vi "RC_STM_Client 3.vi"() -> ()   [LabVIEW 2019, in "RemoteControl.STM.lvclass"]
uses:
  RemoteControl.STM.lvclass
  RemoteControl/RemoteControl.lvclass
  <userlib>/_OpenG.lib/numeric/numeric.llb/Random Number Within Range - I32__ogtk.vi
  <userlib>/_OpenG.lib/error/error.llb/Filter Error Codes (Array)__ogtk.vi
panel:
  in  "milliseconds to wait":u32
  out "time (1 message) (ms)":u32
  out "startup time (ms)":u32
  out "messsages/s":dbl
  in  "remote port":u16=6341
  in  "address":string
  out "Data reponse":string
  out "Messages":i32
  in  "Stop":bool
  out "Command reponse":string
  out "Command":string
  out "meta data\n(available commands)":string
  out "error out":errorcluster
  # "CLIENT (API)"
  # "Connection info"
  # "Message Sent"
  # "Message Received"
  # "Metrics"
  # "3"
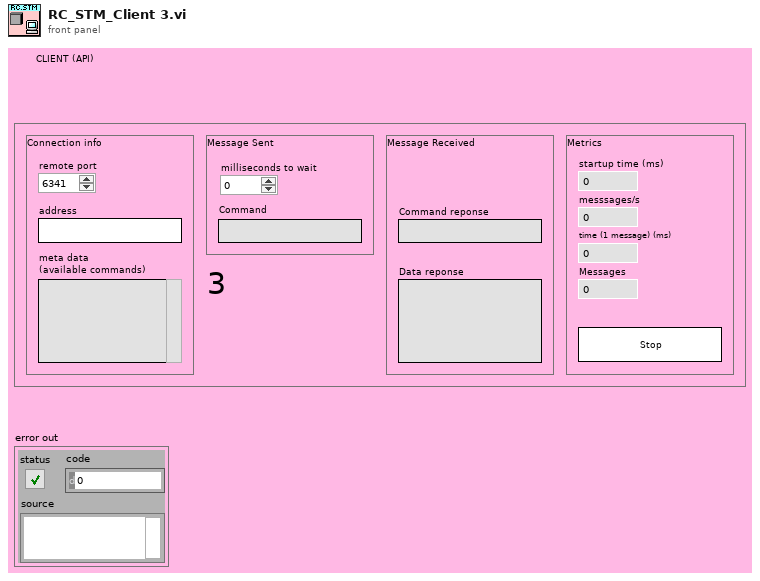
[diagram p1: front panel]
types:
  T1 = typedef "NI STM.lvlib/MetaDataElement.ctl" = string
  T2 = cluster{"Command out":string, "Data out":variant, string}
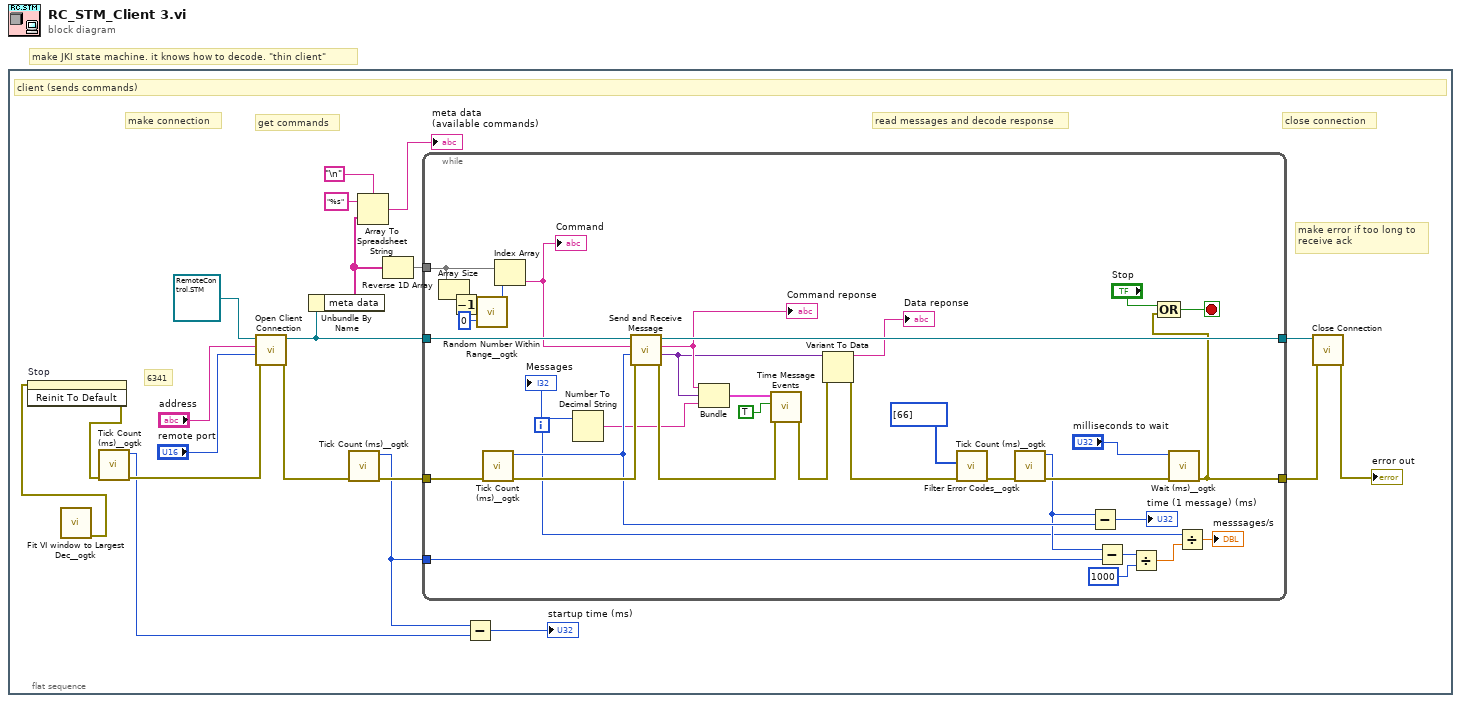
[diagram p0: block diagram]
diagram:
  # "make JKI state machine. it knows how to decode. \"thin client\""
  n1 = flat-sequence {
    frame #0 {
      # "close connection"
      # "read messages and decode response"
      # "get commands"
      # "make connection"
      # "6341"
      # "make error if too long to\nreceive ack"
      # "client (sends commands)"
      n2 = call <userlib>:"Fit VI window to Largest Dec__ogtk.vi"() -> ("error out"=w2:errorcluster)  [unwired: 6 in, 1 out]
      n3 = invoke on="Stop" class="Bool" method="Reinit To Default"(error in=w2) -> (error out=w18:errorcluster)  [unwired: 2 in, 2 out]
      n4 = call <userlib>:"Tick Count (ms)__ogtk.vi"("error in (no error)"=w18) -> ("error out"=w12:errorcluster, "millisecond timer value"=w8:u32)  [unwired: 9 in]
      n5 = call-dynamic "Open Client Connection.vi"("error in (no error)"=w12, "Port"="remote port", "address"="address", "RemoteControl.STM in"=refnum<class "RemoteControl.STM.lvclass"> refnum) -> ("error out"=w11:errorcluster, "RemoteControl.STM out"=w17:refnum<class "RemoteControl.STM.lvclass">)  [unwired: 6 in]
      n6 = Unbundle By Name(w17) -> ("meta data"=w6:T1[])
      n7 = call <userlib>:"Tick Count (ms)__ogtk.vi"("error in (no error)"=w11) -> ("error out"=w10:errorcluster, "millisecond timer value"=w1:u32)  [unwired: 9 in]
      n8 = Array To Spreadsheet String(delimiter (Tab)="\n", array=w6, 3:"%s" ("format string")) -> (spreadsheet string=→"meta data\n(available commands)":string)
      n9 = Reverse 1D Array(array=w6) -> (reversed array=w14:T1[])
      n10 = while {
        tunnel: [w32] -> w20
        tunnel: [w52] -> w19
        tunnel: w10 -> [w47]
        tunnel: w17 -> [w53]
        tunnel: w14 -> [w36]
        tunnel: w1 -> [w23]
        i -> [w22]
        stop <- w55 stop-if-true
        n11 = Array Size(array=w36) -> (size(s)=w37:i32)
        n12 = Decrement(x=w37) -> (x-1=w35:i32)
        n13 = call-poly <userlib>:"Random Number Within Range__ogtk.vi"("High"=w35, "Low"=0) -> ("Random Number"=w39:i32)  [unwired: 3 in]
        n14 = call <userlib>:"Tick Count (ms)__ogtk.vi"("error in (no error)"=w47) -> ("error out"=w46:errorcluster, "millisecond timer value"=w33:u32)  [unwired: 9 in]
        n15 = Index Array(array=w36, index=w39) -> (element=w48:T1)
        "Command" <- w48
        n16 = Number To Decimal String(number=w22) -> (decimal integer string=w21:string)  [unwired: 1 in]
        n17 = call-dynamic "Send and Receive Message.vi"("error in (no error)"=w46, "Data"=w33, "Command"=w48, "RemoteControl in"=w53) -> ("error out"=w34:errorcluster, "Data out"=w31:variant, "Command out"=w45:string, "RemoteControl out"=w52:refnum<class "RemoteControl.STM.lvclass">)  [unwired: 4 in]
        "Command reponse" <- w45
        n18 = Bundle("Command out"=w45, "Data out"=w31, w21) -> (w44:T2)  [unwired: 1 in]
        n19 = call "Time Message Events.vi"("error in (no error)"=w34, "Debug Mode"=TRUE, "Message in"=w44) -> ("error out"=w30:errorcluster)  [unwired: 6 in, 2 out]
        n20 = Variant To Data(error in=w30, Variant=w31) -> (data=→"Data reponse":string, error out=w29:errorcluster)  [unwired: 1 in]
        n21 = call-poly <userlib>:"Filter Error Codes__ogtk.vi"("Error In"=w29, "Error Codes to Filter"=i32[] [66]) -> ("Error Out"=w51:errorcluster)  [unwired: 7 in, 2 out]
        n22 = call <userlib>:"Tick Count (ms)__ogtk.vi"("error in (no error)"=w51) -> ("error out"=w42:errorcluster, "millisecond timer value"=w25:u32)  [unwired: 9 in]
        n23 = Subtract(x=w25, y=w33) -> (x-y=→"time (1 message) (ms)":u32)
        n24 = Subtract(x=w25, y=w23) -> (x-y=w24:u32)
        n25 = Divide(x=w24, y=u32 1000) -> (x/y=w50:dbl)
        n26 = call <userlib>:"Wait (ms)__ogtk.vi"("error in (no error)"=w42, "milliseconds to wait"="milliseconds to wait") -> ("error out"=w32:errorcluster)  [unwired: 8 in, 1 out]
        n27 = Compound Arithmetic op=OR("Stop", w32) -> (w55:bool)
        n28 = Divide(x=w22, y=w50) -> (x/y=→"messsages/s":dbl)
        "Messages" <- w22
      }
      n29 = Subtract(x=w1, y=w8) -> (x-y=→"startup time (ms)":u32)
      n30 = call-dynamic "Close Connection.vi"("error in (no error)"=w20, "RemoteControl.STM in"=w19) -> ("error out"=→"error out":errorcluster)  [unwired: 8 in, 1 out]
    }
  }
